vi "in_2d interp prepare arrays.vi"(0 "size of Z":i32[](array[numeric]), 5 "X":dbl[][](array[numeric]), 7 "Y":dbl[][](array[numeric]), 9 "xi size":i32[](array[numeric]), 11 "yi size":i32[](array[numeric]), 12 "ntimes":i32=1) -> (3 "new size of Z":i32[](array[numeric]), 4 "X-out":dbl[](array[numeric]), 6 "Y-out":dbl[](array[numeric]), 14 "ntimes remaining":i32=1, 15 "error":i32)   [LabVIEW 2017, in "NI_Gmath.lvlib"]
uses:
  NI_Gmath.lvlib
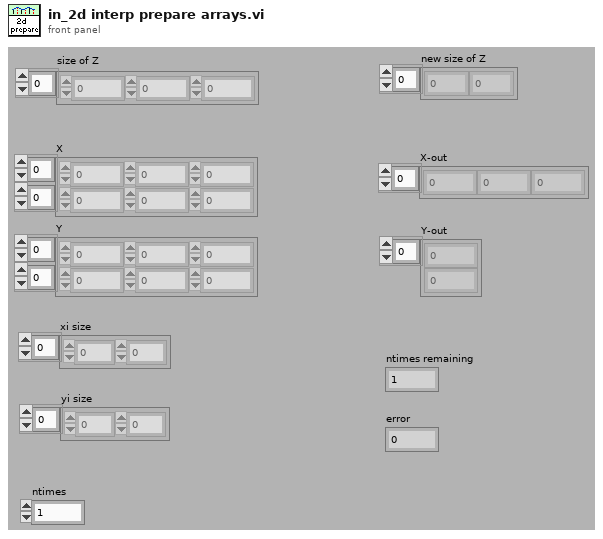
[diagram p1: front panel]
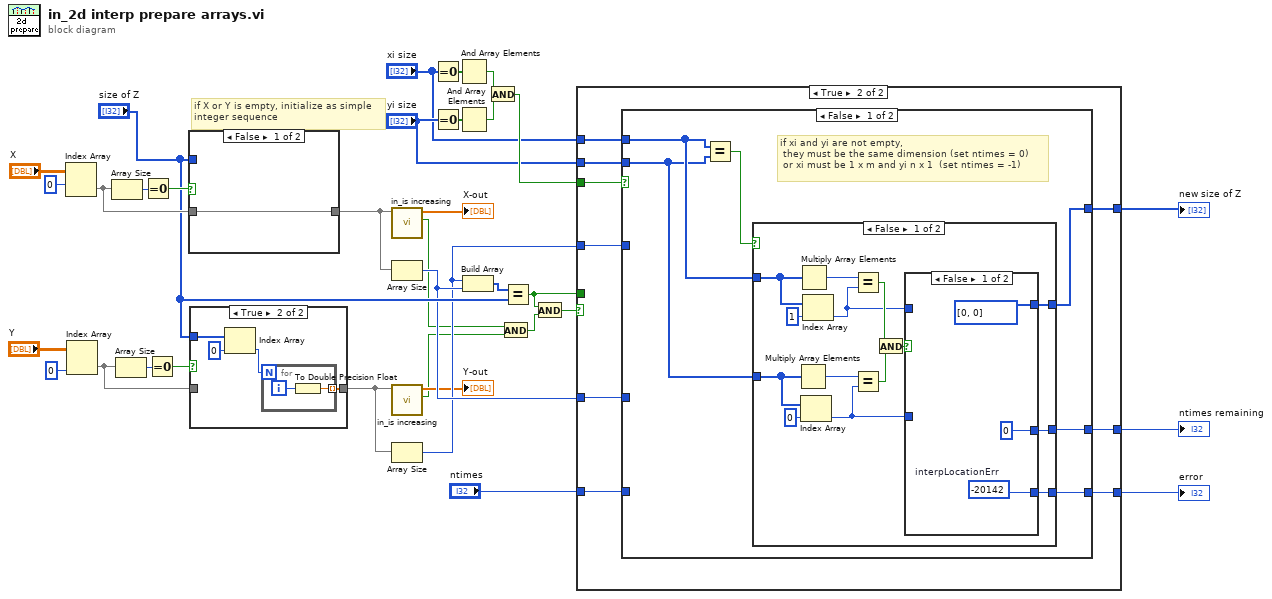
[diagram p0: block diagram]
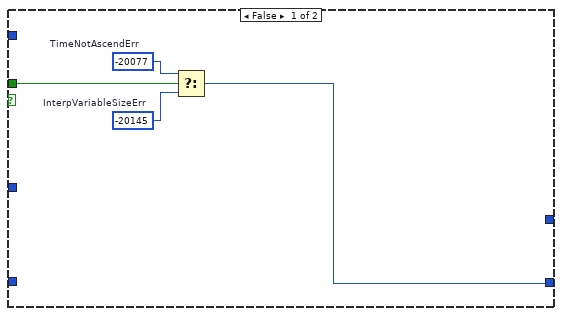
[diagram p2: hidden frame]
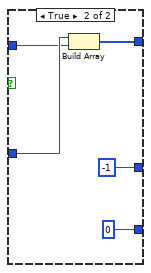
[diagram p3: hidden frame]
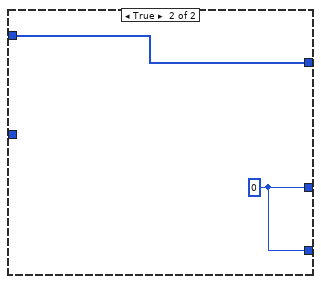
[diagram p4: hidden frame]
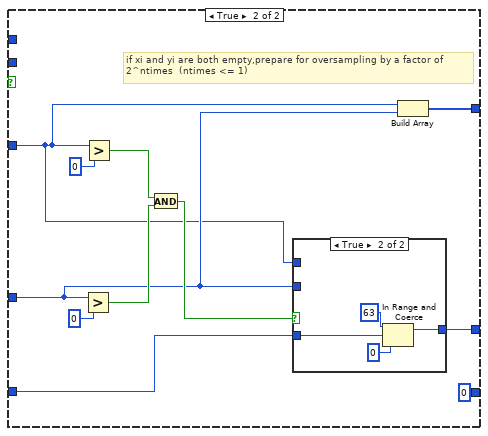
[diagram p5: hidden frame]
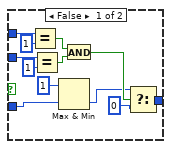
[diagram p6: hidden frame]
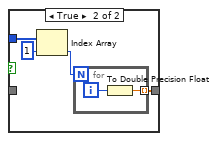
[diagram p8: hidden frame]
diagram:
  # "if X or Y is empty, initialize as simple\ninteger sequence"
  n1 = Index Array(array="X", index (row)=0) -> (element=w31:dbl[])  [unwired: 1 in]
  n2 = Index Array(array="Y", index (col)=0 ("index (row)")) -> (element=w26:dbl[])  [unwired: 1 in]
  n3 = Array Size(array=w31) -> (size(s)=w30:i32)
  n4 = Array Size(array=w26) -> (size(s)=w28:i32)
  n5 = Equal To 0?(x=w30) -> (x = 0?=w29:bool)
  n6 = Equal To 0?(x=w28) -> (x = 0?=w27:bool)
  n7 = case shown="False" w29 {
    tunnel: w31 -> [w35 _]
    tunnel: [w35 w38] -> w9
    tunnel: "size of Z" -> [_ w37]
    frame False {
    }
    frame True {
      n8 = Index Array(array=w37, index=1 ("index (row)")) -> (element=w36:i32)
      n9 = for {
        N: w36 -> [_]
        tunnel: [w40] -> w38 mode=indexing
        i -> [w41]
        n10 = To Double Precision Float(number=w41) -> (double precision float=w40:dbl)
      }
    }
  }
  n11 = case shown="True" w27 {
    tunnel: w26 -> [w42 _]
    tunnel: [w42 w46] -> w7
    tunnel: "size of Z" -> [_ w45]
    frame False {
    }
    frame True {
      n12 = Index Array(array=w45, index=0 ("index (row)")) -> (element=w43:i32)
      n13 = for {
        N: w43 -> [_]
        tunnel: [w47] -> w46 mode=indexing
        i -> [w48]
        n14 = To Double Precision Float(number=w48) -> (double precision float=w47:dbl)
      }
    }
  }
  n15 = call "in_is increasing.vi"("X"=w9) -> ("is increasing"=w4:bool, "X dup"=→"X-out":dbl[])  [unwired: 9 in]
  n16 = Array Size(array=w9) -> (size(s)=w11:i32)
  n17 = call "in_is increasing.vi"("X"=w7) -> ("is increasing"=w5:bool, "X dup"=→"Y-out":dbl[])  [unwired: 9 in]
  n18 = Array Size(array=w7) -> (size(s)=w10:i32)
  n19 = Equal To 0?(x="xi size") -> (x = 0?=w25:bool[])
  n20 = Equal To 0?(x="yi size") -> (x = 0?=w24:bool[])
  n21 = And Array Elements(Boolean array=w25) -> (logical AND=w22:bool)
  n22 = And Array Elements(Boolean array=w24) -> (logical AND=w21:bool)
  n23 = Build Array(w10, w11) -> (w12:i32[])
  n24 = And(x=w22, y=w21) -> (x .and. y?=w20:bool)
  n25 = And(x=w4, y=w5) -> (x .and. y?=w2:bool)
  n26 = Equal?(x=w12, y="size of Z") -> (x = y?=w1:bool)
  n27 = And(x=w1, y=w2) -> (x .and. y?=w3:bool)
  n28 = case shown="True" w3 {
    tunnel: w20 -> [_ w61]
    tunnel: "ntimes" -> [_ w60]
    tunnel: [_ w59] -> w18
    tunnel: w10 -> [_ w58]
    tunnel: w11 -> [_ w57]
    tunnel: [w50 w56] -> w17
    tunnel: "yi size" -> [_ w55]
    tunnel: "xi size" -> [_ w54]
    tunnel: [_ w53] -> w14
    tunnel: w1 -> [w52 _]
    frame False {
      w49 = -20145  # InterpVariableSizeErr
      w51 = -20077  # TimeNotAscendErr
      n29 = Select(t=w51, s=w52, f=w49) -> (s? t:f=w50:i32)
    }
    frame True {
      n30 = case shown="False" w61 {
        tunnel: w60 -> [_ w99]
        tunnel: [w66 w102] -> w59
        tunnel: w58 -> [_ w93]
        tunnel: w57 -> [_ w94]
        tunnel: [w65 0 ("error")] -> w56
        tunnel: w55 -> [w63 _]
        tunnel: w54 -> [w64 _]
        tunnel: [w62 w92] -> w53
        frame False {
          # "if xi and yi are not empty,\n they must be the same dimension (set ntimes = 0)\n or xi must be 1 x m and yi n x 1  (set ntimes = -1)"
          n31 = Equal?(x=w64, y=w63) -> (x = y?=w67:bool)
          n32 = case shown="False" w67 {
            tunnel: [w73 w91] -> w66
            tunnel: [w74 w91] -> w65
            tunnel: w64 -> [w75 w90]
            tunnel: w63 -> [w70 _]
            tunnel: [w72 w90] -> w62
            frame False {
              n33 = Multiply Array Elements(1:w70) -> (0:w79:i32)
              n34 = Multiply Array Elements(1:w75) -> (0:w80:i32)
              n35 = Index Array(array=w70, index=0) -> (element=w69:i32)
              n36 = Index Array(array=w75, index=1) -> (element=w68:i32)
              n37 = Equal?(x=w80, y=w68) -> (x = y?=w78:bool)
              n38 = Equal?(x=w79, y=w69) -> (x = y?=w77:bool)
              n39 = And(x=w78, y=w77) -> (x .and. y?=w76:bool)
              n40 = case shown="False" w76 {
                tunnel: [w82 0 ("t")] -> w74
                tunnel: [0 ("t") -1] -> w73
                tunnel: [i32[] [0, 0] ("new size of Z") w85] -> w72
                tunnel: w69 -> [_ w87]
                tunnel: w68 -> [_ w86]
                frame False {
                  w82 = -20142  # interpLocationErr
                }
                frame True {
                  n41 = Build Array(w87, w86) -> (w85:i32[])
                }
              }
            }
            frame True {
              w91 = 0 ("upper limit")
            }
          }
        }
        frame True {
          # "if xi and yi are both empty,prepare for oversampling by a factor of\n2^ntimes  (ntimes <= 1)"
          n42 = Greater?(x=w94, y=0 ("upper limit")) -> (0:w96:bool)
          n43 = Greater?(x=w93, y=0 ("upper limit")) -> (0:w97:bool)
          n44 = And(x=w97, y=w96) -> (x .and. y?=w98:bool)
          n45 = case shown="True" w98 {
            tunnel: [w107 w116] -> w102
            tunnel: w99 -> [w103 w115]
            tunnel: w93 -> [w113 _]
            tunnel: w94 -> [w110 _]
            frame False {
              n46 = Equal?(x=w113, y=1) -> (x = y?=w109:bool)
              n47 = Equal?(x=w110, y=1) -> (x = y?=w108:bool)
              n48 = Max & Min(x=1 ("t"), y=w103) -> (min(x,y)=w104:i32)  [unwired: 1 out]
              n49 = And(x=w109, y=w108) -> (x .and. y?=w106:bool)
              n50 = Select(t=w104, s=w106, f=0 ("upper limit")) -> (s? t:f=w107:i32)
            }
            frame True {
              n51 = In Range and Coerce(upper limit=63, x=w115, lower limit=0 ("upper limit")) -> (coerced(x)=w116:i32)  [unwired: 1 out]
            }
          }
          n52 = Build Array(w93, w94) -> (w92:i32[])
        }
      }
    }
  }
  "ntimes remaining" <- w18
  "new size of Z" <- w14
  "error" <- w17
